vi "write_read_json text step array.vi"(8 "error in":errorcluster, 10 "json_array_from_file":T1[](array[typedef])=[{"VISA resource name"="", "data num"=0.0, "step_description (prompt)"="(prompt)", "step_json"="", "save results"=FALSE, "step_type"=enum."prompt", "Step_name"="", "data bool"=FALSE}, {"VISA resource name"="", "data num"=1000.0, "step_description (prompt)"="set hipot Voltage", "step_json"="", "save results"=FALSE, "step_type"=enum."set_hipot_V", "Step_name"="", "data bool"=FALSE}, {"VISA resource name"="", "data num"=0.0, "step_description (prompt)"="read hipot v", "step_json"="", "save results"=FALSE, "step_type"=enum."read_hipot_V", "Step_name"="", "data bool"=FALSE}] {"data num" format="%.2f"}, 11 "write_read":T3=enum."read") -> (0 "error out":errorcluster, 2 "steps array out":T1[](array[typedef]) {"data num" format="%.2f"})   [LabVIEW 2020]
uses:
  controls/step.ctl
  controls/step_type.ctl
  controls/write_read.ctl
  3e47bdee-b09f-426d-96e8-78c270cf6aec.vi
  <vilib>/JDP Science/JSONtext/JSON text to Variant.vi
  <vilib>/JDP Science/JSONtext/JSONtext.lvlib
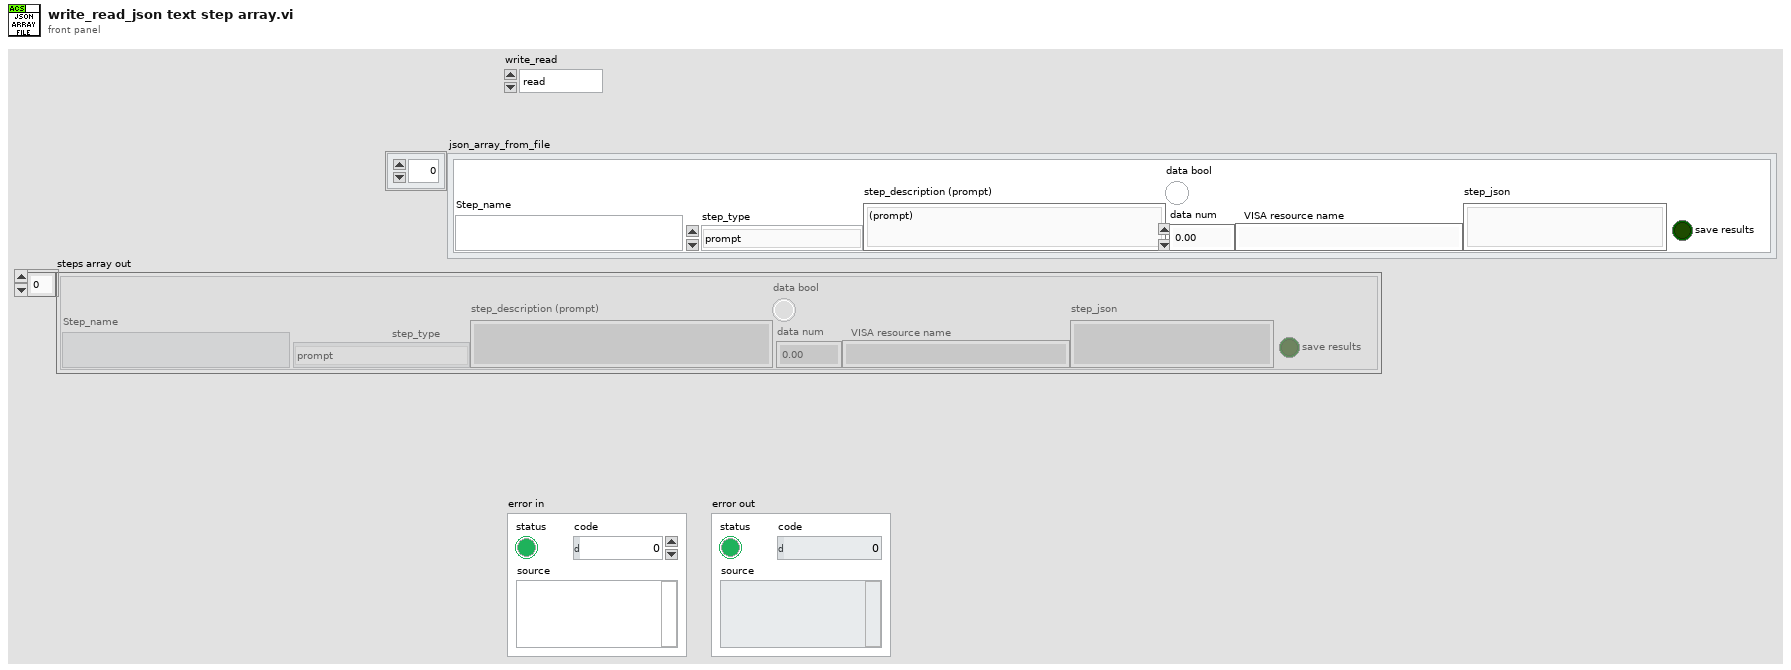
[diagram p1: front panel]
types:
  T1 = typedef "step.ctl" = cluster{"VISA resource name":string, "data num":dbl, "step_description (prompt)":string, "step_json":string, "save results":bool, "step_type":T2, "Step_name":string, "data bool":bool}
  T2 = typedef "step_type.ctl" = enum16{"default", "init", "start test", "prompt", "sequence#", "12V power supply on_off", "set_hipot_V", "set_hipot_I_limit", "set_hipot_ramping (sec)", "set hipot_hold_time", "read_hipot_V", "read_hipot_I", "set_daq", "read_daq", "flash uds", "wait", "record_pass_fail", "error_exit", "exit_program"}
  T3 = typedef "write_read.ctl" = enum16{"write", "read"}
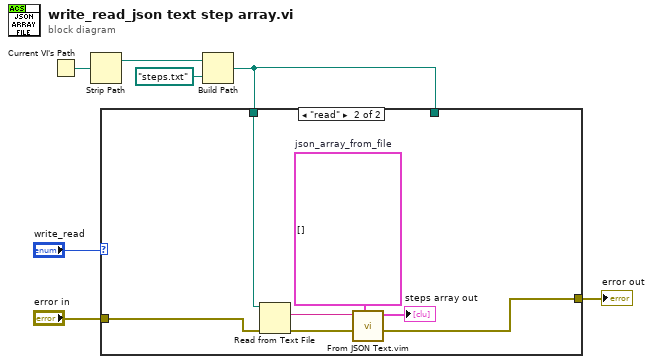
[diagram p0: block diagram]
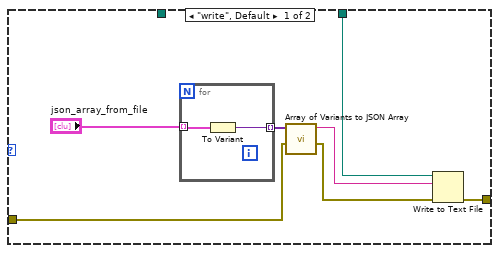
[diagram p2: hidden frame]
diagram:
  n1 = Current VI's Path() -> (path=w7:path)
  n2 = Strip Path(path=w7) -> (stripped path=w6:path)  [unwired: 1 out]
  n3 = Build Path(base path=w6, name or relative path=path "steps.txt") -> (appended path=w1:path)
  n4 = case shown="\"read\"" "write_read" {
    tunnel: w1 -> [w12 _]
    tunnel: "error in" -> [w10 w20]
    tunnel: [w8 w17] -> w2
    tunnel: w1 -> [_ w19]
    frame "write", Default {
      n5 = for {
        tunnel: "json_array_from_file" -> [w15] mode=indexing
        tunnel: [w16] -> w14 mode=indexing
        n6 = To Variant(anything=w15) -> (Variant=w16:variant)
      }
      n7 = call <vilib>:"Array of Variants to JSON Array.vi"("error in (no error)"=w10, "Array of Variants"=w14) -> ("error out"=w9:errorcluster, "<JSON>"=w13:string)  [unwired: 8 in]
      n8 = Write to Text File(file (use dialog)=w12, text=w13, error in=w9) -> (error out=w8:errorcluster)  [unwired: 1 in, 2 out]
    }
    frame "read" {
      w21 = T1[] []  # json_array_from_file
      n9 = Read from Text File(file (use dialog)=w19, error in=w20) -> (text=w22:string, error out=w18:errorcluster)  [unwired: 2 in, 2 out]
      n10 = call "From JSON Text.vim"("Data Type and Default Value"=w21, "error in (no error)"=w18, "JSON"=w22) -> ("error out"=w17:errorcluster, "Data out"=→"steps array out":T1[])  [unwired: 7 in]
    }
  }
  "error out" <- w2
